vi "fp4task1.vi"   [LabVIEW 2016]
uses:
  <vilib>/NXT/Block Support/NXT_InputPort.ctl
  <vilib>/NXT/Block Support/NXT_OutputPort.ctl
  <vilib>/NXT/NXTIO Xnodes/NXTIONodeSubVIs/LEGOResetMotors.vi
  <vilib>/NXT/Dual Mode Library/Waits/Wait_Bump.vi
  <vilib>/NXT/Dual Mode Library/Sensors/EV3_Color_Reflect.vi
  <vilib>/NXT/Dual Mode Library/Sensors/Touch_Pressed.vi
  <vilib>/NXT/NXTIO Xnodes/NXTIONodeSubVIs/NXTMoveMotors.vi
  <vilib>/NXT/NXTIO Xnodes/NXTIONodeSubVIs/NXTMotorRunDistance.vi
  <vilib>/NXT/NXTIO Xnodes/NXTIONodeSubVIs/LEGOStopAllMotors.vi
  <vilib>/NXT/Dual Mode Library/Sound/Tone.vi
  <vilib>/NXT/Dual Mode Library/Waits/Wait_Num.vi
  <vilib>/NXT/Dual Mode Library/Sound/PlayA.vi
  <vilib>/NXT/Subs/LVHSConnector.ctl
  <vilib>/NXT/NXTIO Xnodes/AddressXNode/NXTIOAddress.xnode
  <vilib>/NXT/NXTIO Xnodes/NXTIOXNode/NXTIO.xnode
  <vilib>/NXT/LegoClasses/BrickReference/BrickReference.lvclass
types:
  T1 = typedef "NXT_OutputPort.ctl" = u8
  T2 = typedef "NXT_InputPort.ctl" = u32
  T3 = typedef "LVHSConnector.ctl" = refnum<class "BrickReference.lvclass">
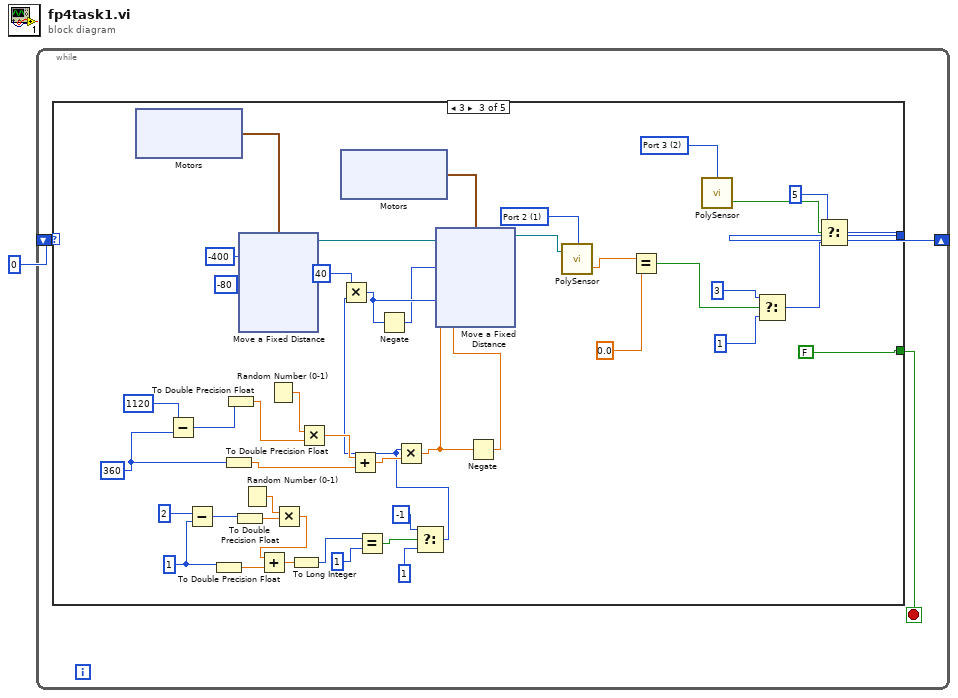
[diagram p0: block diagram]
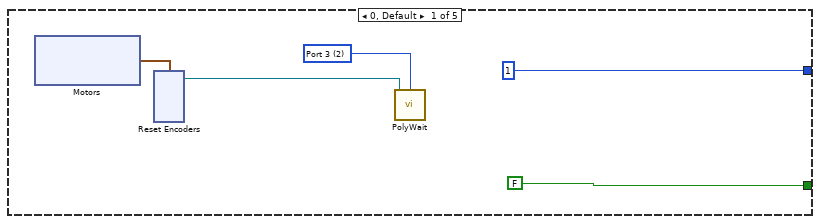
[diagram p2: hidden frame]
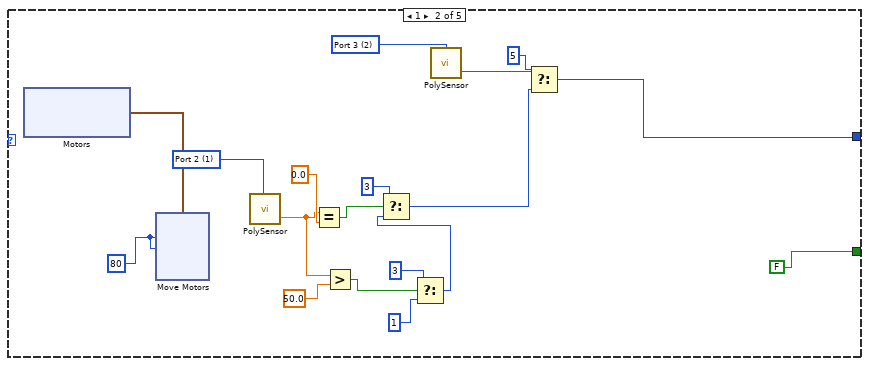
[diagram p3: hidden frame]
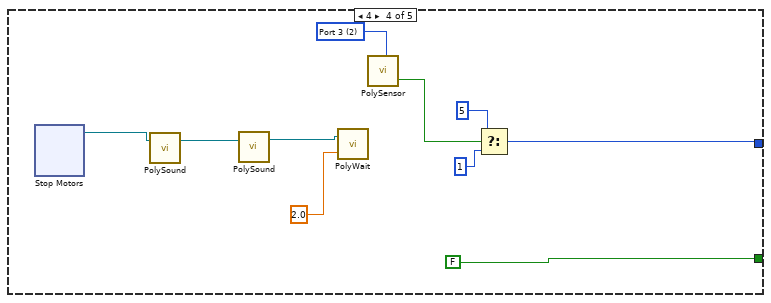
[diagram p4: hidden frame]
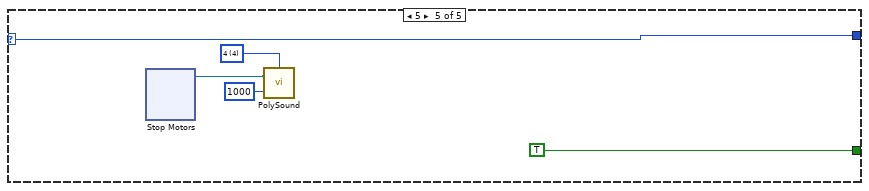
[diagram p5: hidden frame]
diagram:
  n1 = while {
    shift-right: [w4] -> _
    shift-left: 0 -> [w3]
    stop <- w2 stop-if-true
    n2 = case shown="3" w3 {
      selector: w3 -> [_ _ _ _ w130]
      tunnel: [1 w29 w86 w115 w130] -> w4
      tunnel: [FALSE FALSE FALSE FALSE TRUE] -> w2
      frame 0, Default {
        w6 = T2 2 items=["Port 1", "Port 2", "Port 3", "Port 4"] ("Port (Port 1)")
        n3 = xnode "Motors"() -> ("Motor"=w9:cluster{"Port":T1, "Port":T1})
        n4 = xnode "Reset Encoders"("Motors"=w9) -> ("NXT/EV3"=w5:T3)  [unwired: 1 in]
        n5 = call-poly <vilib>:"PolyWait.vi"("NXT/EV3"=w5, "Port (Port 1)"=w6) -> ()  [unwired: 2 in, 1 out]
      }
      frame 1 {
        w15 = 80 ("Distance 1")
        w25 = T2 2 items=["Port 1", "Port 2", "Port 3", "Port 4"] ("Port (Port 1)")
        w26 = T2 1 items=["Port 1", "Port 2", "Port 3", "Port 4"] ("Port (Port 1)")
        n6 = xnode "Motors"() -> ("Motor"=w16:cluster{"Port":T1, "Port":T1})
        n7 = xnode "Move Motors"("Power/Speed 2"=w15, "Power/Speed 1"=w15, "Motors"=w16) -> ()  [unwired: 1 in, 1 out]
        n8 = call-poly <vilib>:"PolySensor.vi"("Port (Port 1)"=w26) -> ("Scaled Value"=w22:sgl)  [unwired: 2 in, 1 out]
        n9 = Equal?(x=w22, y=sgl 0.0) -> (x = y?=w32:bool)
        n10 = Greater?(x=w22, y=sgl 50.0) -> (0:w20:bool)
        n11 = Select(t=3, s=w20, f=1) -> (s? t:f=w17:i32)
        n12 = Select(t=3, s=w32, f=w17) -> (s? t:f=w23:i32)
        n13 = call-poly <vilib>:"PolySensor.vi"("Port (Port 1)"=w25) -> ("Yes / No"=w24:bool)  [unwired: 2 in, 1 out]
        n14 = Select(t=5, s=w24, f=w23) -> (s? t:f=w29:i32)
      }
      frame 3 {
        w59 = 1
        w66 = 360
        w72 = -80 ("Distance 1")
        w73 = -400 ("Distance 1")
        w77 = T2 1 items=["Port 1", "Port 2", "Port 3", "Port 4"] ("Port (Port 1)")
        w79 = T2 2 items=["Port 1", "Port 2", "Port 3", "Port 4"] ("Port (Port 1)")
        n15 = xnode "Motors"() -> ("Motor"=w74:cluster{"Port":T1, "Port":T1})
        n16 = Subtract(x=1120, y=w66) -> (x-y=w67:i32)
        n17 = Subtract(x=2, y=w59) -> (x-y=w60:i32)
        n18 = To Double Precision Float(number=w59) -> (double precision float=w58:dbl)
        n19 = To Double Precision Float(number=w66) -> (double precision float=w62:dbl)
        n20 = To Double Precision Float(number=w67) -> (double precision float=w65:dbl)
        n21 = To Double Precision Float(number=w60) -> (double precision float=w57:dbl)
        n22 = xnode "Move a Fixed Distance"("Speed 2"=w72, "Speed 1"=w72, "Distance 2"=w73, "Distance 1"=w73, "Motors"=w74) -> ("NXT/EV3"=w71:T3)  [unwired: 1 in]
        n23 = Random Number (0-1)() -> (number: 0 to 1=w56:dbl)
        n24 = Random Number (0-1)() -> (number: 0 to 1=w64:dbl)
        n25 = Multiply(x=w56, y=w57) -> (x*y=w54:dbl)
        n26 = Add(x=w54, y=w58) -> (x+y=w55:dbl)
        n27 = To Long Integer(number=w55) -> (32bit integer=w52:i32)
        n28 = Multiply(x=w64, y=w65) -> (x*y=w63:dbl)
        n29 = xnode "Motors"() -> ("Motor"=w75:cluster{"Port":T1, "Port":T1})
        n30 = Add(x=w63, y=w62) -> (x+y=w48:dbl)
        n31 = Equal?(x=w52, y=1) -> (x = y?=w51:bool)
        n32 = Select(t=-1, s=w51, f=1) -> (s? t:f=w44:i32)
        n33 = Multiply(x=40 ("Distance 1"), y=w44) -> (x*y=w43:i32)
        n34 = Negate(x=w43) -> (-x=w42:i32)
        n35 = Multiply(x=w44, y=w48) -> (x*y=w45:dbl)
        n36 = Negate(x=w45) -> (-x=w46:dbl)
        n37 = xnode "Move a Fixed Distance"("Speed 2"=w43, "Speed 1"=w42, "Distance 2"=w45, "Distance 1"=w46, "Motors"=w75, "NXT/EV3"=w71) -> ("NXT/EV3"=w69:T3)
        n38 = call-poly <vilib>:"PolySensor.vi"("NXT/EV3"=w69, "Port (Port 1)"=w77) -> ("Scaled Value"=w76:sgl)  [unwired: 1 in, 1 out]
        n39 = Equal?(x=w76, y=0.0) -> (x = y?=w81:bool)
        n40 = call-poly <vilib>:"PolySensor.vi"("Port (Port 1)"=w79) -> ("Yes / No"=w78:bool)  [unwired: 2 in, 1 out]
        n41 = Select(t=3, s=w81, f=1) -> (s? t:f=w84:i32)
        n42 = Select(t=5, s=w78, f=w84) -> (s? t:f=w86:i32)
      }
      frame 4 {
        w114 = T2 2 items=["Port 1", "Port 2", "Port 3", "Port 4"] ("Port (Port 1)")
        n43 = xnode "Stop Motors"() -> ("NXT/EV3"=w122:T3)  [unwired: 2 in]
        n44 = call-poly <vilib>:"PolySound.vi"("NXT/EV3"=w122) -> ("NXT/EV3"=w121:T3)  [unwired: 3 in]
        n45 = call-poly <vilib>:"PolySound.vi"("NXT/EV3"=w121) -> ("NXT/EV3"=w119:T3)  [unwired: 3 in]
        n46 = call-poly <vilib>:"PolyWait.vi"("Time (1 sec)"=sgl 2.0, "NXT/EV3"=w119) -> ()  [unwired: 2 in, 1 out]
        n47 = call-poly <vilib>:"PolySensor.vi"("Port (Port 1)"=w114) -> ("Yes / No"=w113:bool)  [unwired: 2 in, 1 out]
        n48 = Select(t=5, s=w113, f=1) -> (s? t:f=w115:i32)
      }
      frame 5 {
        w127 = u16 4 items=["3"=3, "4"=4, "5"=5, "6"=6, "7"=7] ("Octave")
        n49 = xnode "Stop Motors"() -> ("NXT/EV3"=w128:T3)  [unwired: 2 in]
        n50 = call-poly <vilib>:"PolySound.vi"("Duration (500 ms)"=u16 1000, "NXT/EV3"=w128, "Octave"=w127) -> ()  [unwired: 1 in, 1 out]
      }
    }
  }
